vi "create_pattern.vi"(8 "error in (no error)":errorcluster, 11 "StimulatorDL090727DAQmx in":refnum<class "StimulatorDL090727Writer.lvclass">) -> (0 "error out":errorcluster, 3 "StimulatorDL090727DAQmx out":refnum<class "StimulatorDL090727Writer.lvclass">)   [LabVIEW 2010, in "StimulatorDL090727Writer.lvclass"]
uses:
  StimulatorDL090727Writer.lvclass
  common/enumerations/functional_global_action_enum.ctl
  StimulatorDL090727Writer.lvclass/StimulatorDL090727Writer.ctl
panel:
  out "stimulation pattern":dbl[](graph)
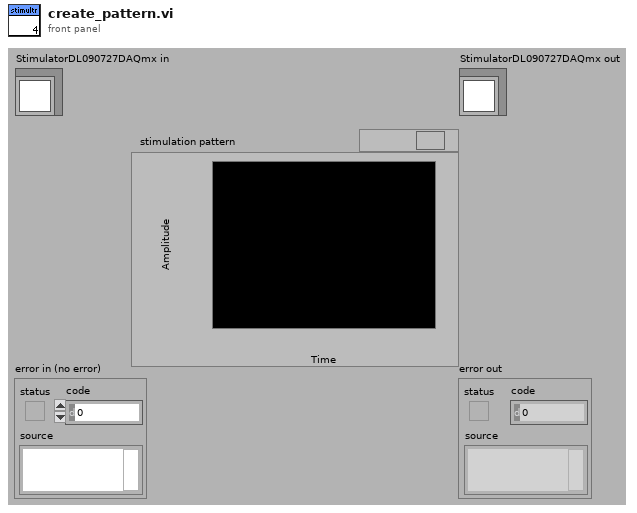
[diagram p1: front panel]
types:
  T1 = typedef "functional_global_action_enum.ctl" = enum16{"get", "set", "reset"}
  T2 = typedef "StimulatorDL090727Writer.lvclass/pattern_enum.ctl" = enum16{"sine wave", "square"}
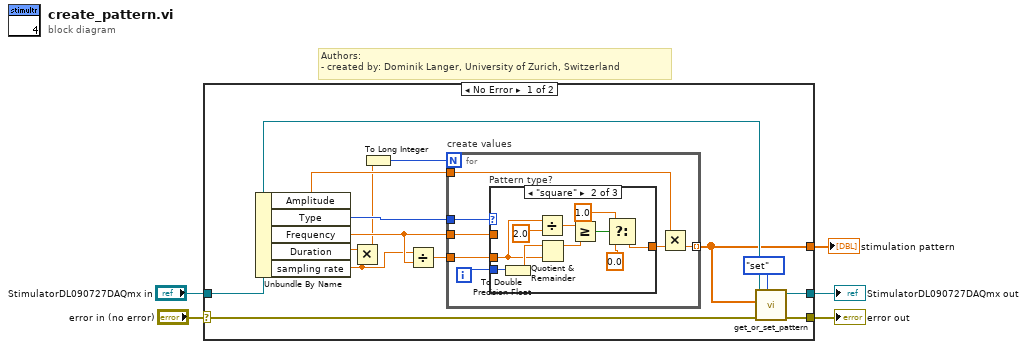
[diagram p0: block diagram]
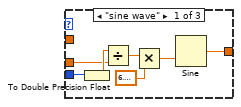
[diagram p2: hidden frame]
diagram:
  # "Authors: \n- created by: Dominik Langer, University of Zurich, Switzerland"
  n1 = case shown="No Error" "error in (no error)" {
    selector: "error in (no error)" -> [w8 w45]
    tunnel: [w15 w45] -> w4
    tunnel: [w14 w44] -> w2
    tunnel: "StimulatorDL090727DAQmx in" -> [w9 w44]
    tunnel: [w6 _] -> w1
    frame No Error {
      n2 = Unbundle By Name(w9) -> ("Amplitude"=w18:dbl, "Type"=w19:T2, "Frequency"=w17:dbl[unit], "Duration"=w12:dbl[unit], "sampling rate"=w7:dbl[unit])
      n3 = Multiply(x=w12, y=w7) -> (x*y=w10:dbl)
      n4 = To Long Integer(number=w10) -> (32bit integer=w11:i32)
      n5 = Divide(x=w7, y=w17) -> (x/y=w16:dbl)
      n6 = for "create values" {
        N: w11 -> [_]
        tunnel: w18 -> [w20]
        tunnel: w19 -> [w26]
        tunnel: [w21] -> w6 mode=indexing
        tunnel: w17 -> [w25]
        tunnel: w16 -> [w23]
        i -> [w24]
        n7 = case "Pattern type?" shown="\"square\"" w26 {
          tunnel: [w33 w35 _] -> w22
          tunnel: w25 -> [_ _ _]
          tunnel: w24 -> [w29 w43 _]
          tunnel: w23 -> [w28 w41 _]
          frame "sine wave" {
            n8 = To Double Precision Float(number=w29) -> (double precision float=w32:dbl)
            n9 = Divide(x=w32, y=w28) -> (x/y=w31:dbl)
            n10 = Multiply(x=w31, y=6.283185307179586) -> (x*y=w27:dbl)
            n11 = Sine(x=w27) -> (sin(x)=w33:dbl)
          }
          frame "square" {
            n12 = To Double Precision Float(number=w43) -> (double precision float=w42:dbl)
            n13 = Divide(x=w41, y=2.0) -> (x/y=w39:dbl)
            n14 = Quotient & Remainder(x=w42, y=w41) -> (x-y*floor(x/y)=w34:dbl)  [unwired: 1 out]
            n15 = Greater Or Equal?(x=w39, y=w34) -> (x >= y?=w38:bool)
            n16 = Select(t=1.0, s=w38, f=0.0) -> (s? t:f=w35:dbl)
          }
          frame Default {
          }
        }
        n17 = Multiply(x=w20, y=w22) -> (x*y=w21:dbl)
      }
      n18 = call-dynamic "get_or_set_pattern.vi"("action"=functional_global_action_enum."set", "error in (no error)"=w8, "samples in"=w6, "Stimulator090724 in"=w9) -> ("error out"=w15:errorcluster, "Stimulator090724 out"=w14:refnum<class "StimulatorDL090727Writer.lvclass">)  [unwired: 6 out]
    }
    frame Error {
    }
  }
  "error out" <- w4
  "StimulatorDL090727DAQmx out" <- w2
  "stimulation pattern" <- w1
